vi "fpga_Channel_fifo_ov.vi"(0 "Main clock":u32, 1 "Scheduler":u8, 2 "Signal IN":bool, 3 "ID":u8, 4 "overflow":bool) -> (5 "32 bit Output":u32, 6 "Timed Out?":bool, 7 "Data Available":bool)   [LabVIEW 2011]
uses:
  <vilib>/rvi/DataTransferAndStorage/Container/Common/niFpgaContainerMetaDataKey.ctl
  <vilib>/rvi/DataTransferAndStorage/Container/Common/niFpgaContainerState.ctl
  <vilib>/rvi/DataTransferAndStorage/Container/Common/niFpgaDataTypeControl.ctl
  <vilib>/rvi/DataTransferAndStorage/Container/Common/niFpgaContainerImplementationControl.ctl
  <vilib>/rvi/DataTransferAndStorage/Container/Common/niFpgaContainerArbitrationOptionsControl.ctl
  <vilib>/rvi/DataTransferAndStorage/Container/Common/niFpgaTransferTypeControl.ctl
  <vilib>/rvi/DataTransferAndStorage/Container/Common/niFpgaContainerInitializationParameters.ctl
  <vilib>/rvi/Memory/Memory_Types/niFpgaMemoryInterfaceConfiguration.ctl
  <vilib>/rvi/FIFO/Fifo_Types/niFpgaFifoControlLogicControl.ctl
  <vilib>/rvi/eio/common/nirviEmuReportErrorAndStop.vi
  <vilib>/rvi/DataTransferAndStorage/Container/Common/niFpgaContainerSetEmuInfo.vi
  <vilib>/rvi/DataTransferAndStorage/Container/Common/niFpgaContainerGetUniqueNameForEmu.vi
  <vilib>/rvi/FIFO/Fifo_Resource/nirvififoEmulationSetSize.vi
  <vilib>/rvi/LocalResourceManager/LocalResourceManager.xnode
  <vilib>/rvi/DataTransferAndStorage/Container/XNode/niFpgaContainer.xnode
  <vilib>/rvi/FIFO/Fifo_Resource/nirvififoEmulationWrite.vi
  <vilib>/rvi/FIFO/Fifo_Resource/nirvififoEmulationRead.vi
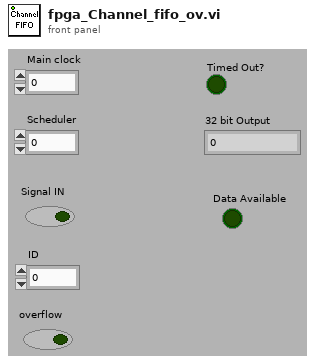
[diagram p1: front panel]
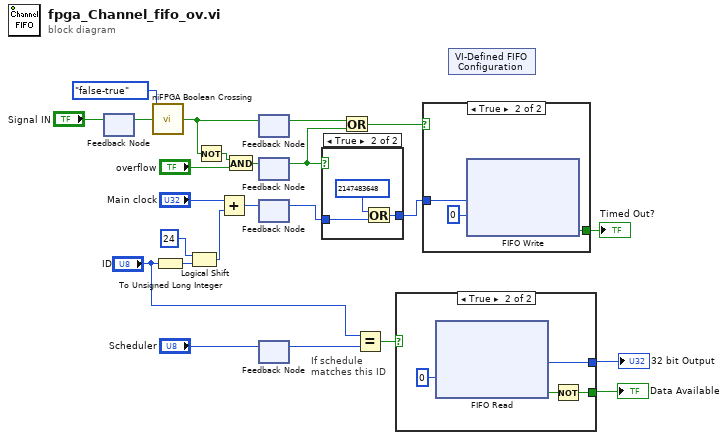
[diagram p0: block diagram]
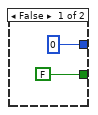
[diagram p3: hidden frame]
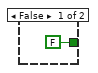
[diagram p4: hidden frame]
diagram:
  # "If schedule \nmatches this ID"
  n1 = feedback #1() -> ()  [unwired: 2 in]
  n2 = feedback-in #1("Signal IN") -> ()
  n3 = call <vilib>:"niFPGA Boolean Crossing.vi"("input"="Signal IN", "direction"=enum8{"either", "false-true", "true-false"}."false-true") -> ("crossing"=w2:bool)  [unwired: 7 in]
  n4 = To Unsigned Long Integer(number="ID") -> (unsigned 32bit integer=w12:u32)
  n5 = Logical Shift(y=i8 24, x=w12) -> (x << y=w13:u32)
  n6 = Not(x=w2) -> (.not. x?=w1:bool)
  n7 = Add(x="Main clock", y=w13) -> (x+y=w14:u32)
  n8 = And(x=w1, y="overflow") -> (x .and. y?=w3:bool)
  n9 = feedback #2() -> (w6:bool)  [unwired: 1 in]
  n10 = feedback-in #2(w2) -> ()
  n11 = feedback #3() -> (w5:bool)  [unwired: 1 in]
  n12 = feedback-in #3(w3) -> ()
  n13 = feedback-in #4(w14) -> ()
  n14 = feedback #4() -> (w18:u32)  [unwired: 1 in]
  n15 = feedback-in #5("Scheduler") -> ()
  n16 = feedback #5() -> (w19:u8)  [unwired: 1 in]
  n17 = case shown="True" w5 {
    tunnel: w18 -> [w24 w27]
    tunnel: [w24 w26] -> w17
    frame False {
    }
    frame True {
      n18 = Or(x=u32 2147483648, y=w27) -> (x .or. y?=w26:u32)
    }
  }
  n19 = Or(x=w6, y=w5) -> (x .or. y?=w7:bool)
  n20 = Equal?(x="ID", y=w19) -> (x = y?=w20:bool)
  n21 = case shown="True" w20 {
    tunnel: [FALSE w30] -> w22
    tunnel: [u32 0 ("Element") w31] -> w23
    frame False {
    }
    frame True {
      n22 = xnode ("FIFO Read")("Timeout"=0) -> ("Element"=w31:u32, "Timed Out?"=w32:bool)  [unwired: 1 in, 1 out]
      n23 = Not(x=w32) -> (.not. x?=w30:bool)
    }
  }
  "32 bit Output" <- w23
  "Data Available" <- w22
  n24 = case shown="True" w7 {
    tunnel: w17 -> [_ w36]
    tunnel: [FALSE ("Timed Out?") w35] -> w8
    frame False {
    }
    frame True {
      n25 = xnode ("FIFO Write")("Element"=w36, "Timeout"=0) -> ("Timed Out?"=w35:bool)  [unwired: 1 in, 1 out]
    }
  }
  "Timed Out?" <- w8
  n26 = xnode "VI-Defined FIFO Configuration"() -> ()  [unwired: 1 out]
